vi "utilities_setTimeMode.vi"(8 "error in (no error)":errorcluster, 10 "time column mode (0: Empty)":T1, 11 "data value":T2={"TargetFile"=path "", "StreamMode"=enum."File", "Append?"=FALSE, "ChunkSize"=0, "TimeColumnMode"=enum."Empty", "TimestampFormat"="", "AbsoluteTime?"=FALSE, "FileAttribute "={"Creator"="", "Title"="", "SheetName"=""}, "Column"=[], "FileRef"=refnum, "MemoryRef"=[], "RecordInfo"=[], " ChannelPreviousInfo"=[], "ChannelFirstRecord"=[], "PredefinedFormattedValueLength"=20, "DiskTemplate"={"XMLRef"=[refnum, refnum, refnum, refnum, refnum, refnum], "ZipPath"=path "", "MetaFile"={"Ref"=refnum, "NextRow"=0, "NextPosition"=0, "Block"=[]}, "TempFolder"=path ""}}) -> (0 "error out":errorcluster, 3 "data value out":T2={"TargetFile"=path "", "StreamMode"=enum."File", "Append?"=FALSE, "ChunkSize"=0, "TimeColumnMode"=enum."Empty", "TimestampFormat"="", "AbsoluteTime?"=FALSE, "FileAttribute "={"Creator"="", "Title"="", "SheetName"=""}, "Column"=[], "FileRef"=refnum, "MemoryRef"=[], "RecordInfo"=[], " ChannelPreviousInfo"=[], "ChannelFirstRecord"=[], "PredefinedFormattedValueLength"=20, "DiskTemplate"={"XMLRef"=[refnum, refnum, refnum, refnum, refnum, refnum], "ZipPath"=path "", "MetaFile"={"Ref"=refnum, "NextRow"=0, "NextPosition"=0, "Block"=[]}, "TempFolder"=path ""}})   [LabVIEW 2020, in "NI_ExcelFile.lvlib"]
uses:
  <vilib>/express/express shared/NI_ExcelFile/NI_ExcelFile.lvlib
  <vilib>/express/express shared/NI_ExcelFile/Ctrls/MainData.ctl
  <vilib>/express/express shared/NI_ExcelFile/Ctrls/StreamMode.ctl
  <vilib>/express/express shared/NI_ExcelFile/Ctrls/TimeColumnMode.ctl
  <vilib>/express/express shared/NI_ExcelFile/Ctrls/FileAttribute.ctl
  <vilib>/express/express shared/NI_ExcelFile/Ctrls/Columns.ctl
  <vilib>/express/express shared/NI_ExcelFile/Ctrls/ColumnInfo.ctl
  <vilib>/express/express shared/NI_ExcelFile/Ctrls/DataType.ctl
  <vilib>/express/express shared/NI_ExcelFile/Ctrls/wd_recordInfo.ctl
  <vilib>/express/express shared/NI_ExcelFile/Ctrls/disk_TemplateFile.ctl
  <vilib>/express/express shared/NI_ExcelFile/Ctrls/meta_file.ctl
  <vilib>/express/express shared/NI_ExcelFile/Ctrls/meta_Block.ctl
  <vilib>/express/express shared/NI_ExcelFile/Ctrls/meta_BlockType.ctl
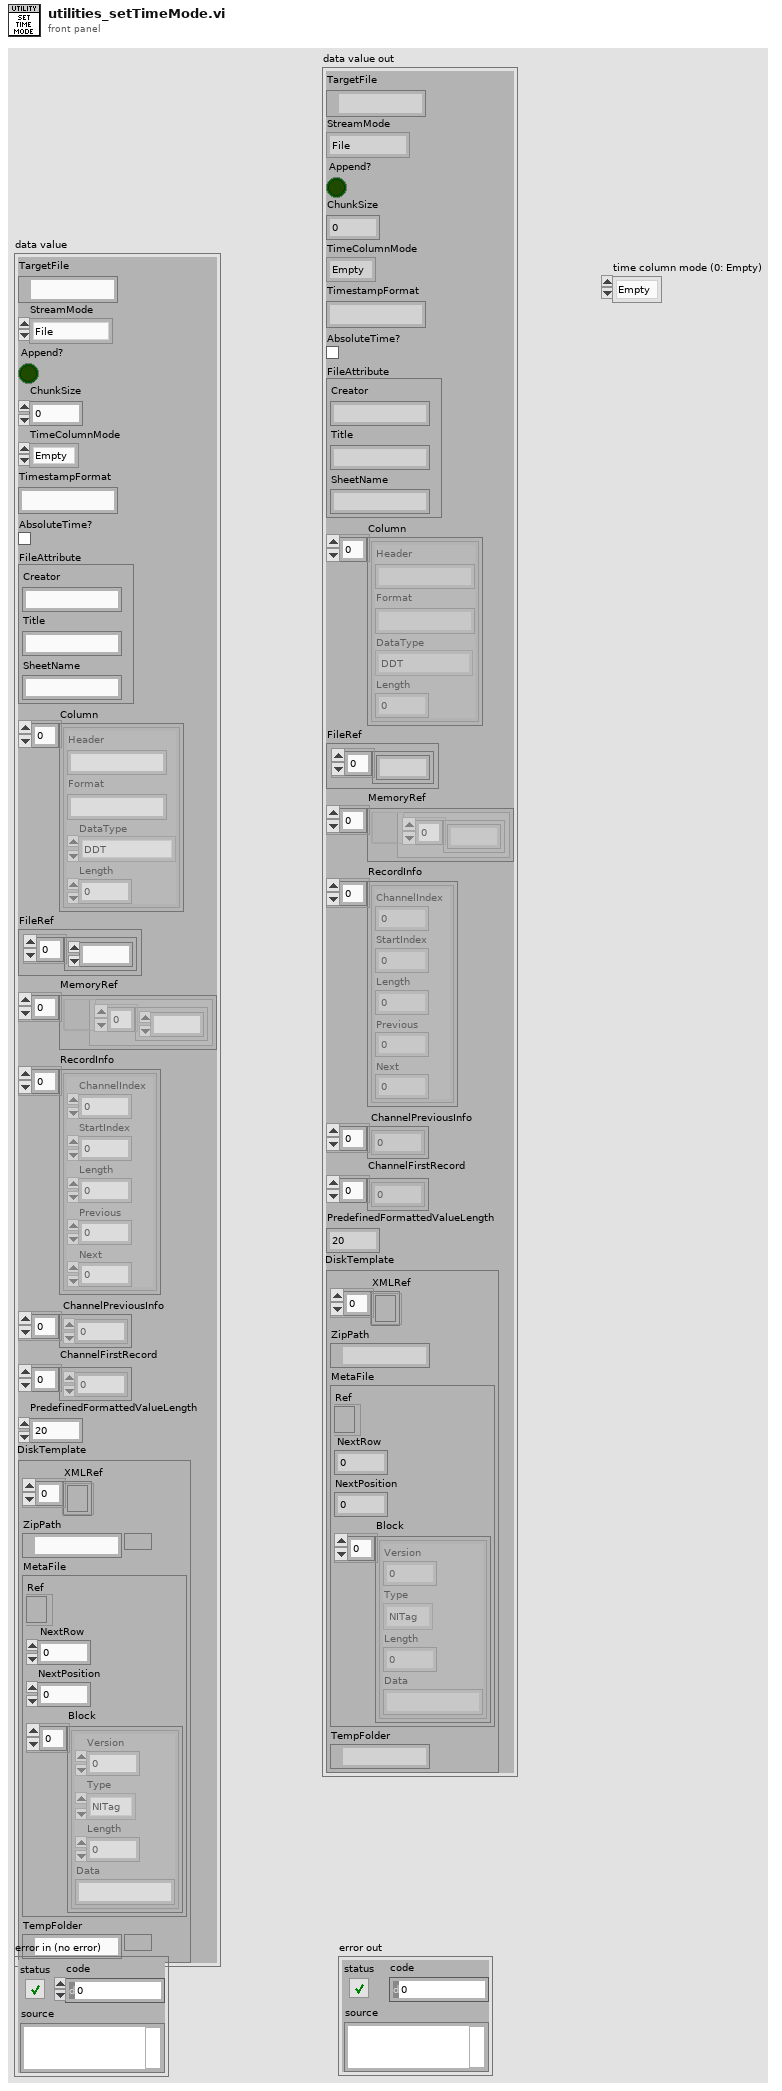
[diagram p1: front panel]
types:
  T1 = typedef "NI_ExcelFile.lvlib/TimeColumnMode.ctl" = enum16{"Empty", "OnePerCh", "One"}
  T2 = typedef "NI_ExcelFile.lvlib/MainData.ctl" = cluster{"TargetFile":path, "StreamMode":T3, "Append?":bool, "ChunkSize":u64, "TimeColumnMode":T1, "TimestampFormat":string, "AbsoluteTime?":bool, "FileAttribute ":T4, "Column":T5, "FileRef":refnum<k1>, "MemoryRef":refnum<data-value>[], "RecordInfo":T8[], " ChannelPreviousInfo":u32[], "ChannelFirstRecord":u32[], "PredefinedFormattedValueLength":i64, "DiskTemplate":T9}
  T3 = typedef "NI_ExcelFile.lvlib/StreamMode.ctl" = enum16{"File", "Memory"}
  T4 = typedef "NI_ExcelFile.lvlib/FileAttribute.ctl" = cluster{"Creator":string, "Title":string, "SheetName":string}
  T5 = typedef "NI_ExcelFile.lvlib/Columns.ctl" = T6[]
  T6 = typedef "NI_ExcelFile.lvlib/ColumnInfo.ctl" = cluster{"Header":string, "Format":string, "DataType":T7, "Length":u64}
  T7 = typedef "NI_ExcelFile.lvlib/DataType.ctl" = enum16{"DDT", "WFM", "Array of STR", "Array of DBL", "Array of I8", "Array of I16", "Array of I32", "Array of I64", "Array of SGL", "Array of U8", "Array of U16", "Array of U32", "Array of U64", "Array of Time"}
  T8 = typedef "NI_ExcelFile.lvlib/wd_recordInfo.ctl" = cluster{"ChannelIndex":u32, "StartIndex":u64, "Length":u64, "Previous":i32, "Next":i32}
  T9 = typedef "NI_ExcelFile.lvlib/disk_TemplateFile.ctl" = cluster{"XMLRef":refnum<file>[], "ZipPath":path, "MetaFile":T10, "TempFolder":path}
  T10 = typedef "NI_ExcelFile.lvlib/meta_file.ctl" = cluster{"Ref":refnum<file>, "NextRow":i32, "NextPosition":i64, "Block":T11[]}
  T11 = typedef "NI_ExcelFile.lvlib/meta_Block.ctl" = cluster{"Version":u16, "Type":T12, "Length":i32, "Data":string}
  T12 = typedef "NI_ExcelFile.lvlib/meta_BlockType.ctl" = enum16{"NITag", "File", "Column"}
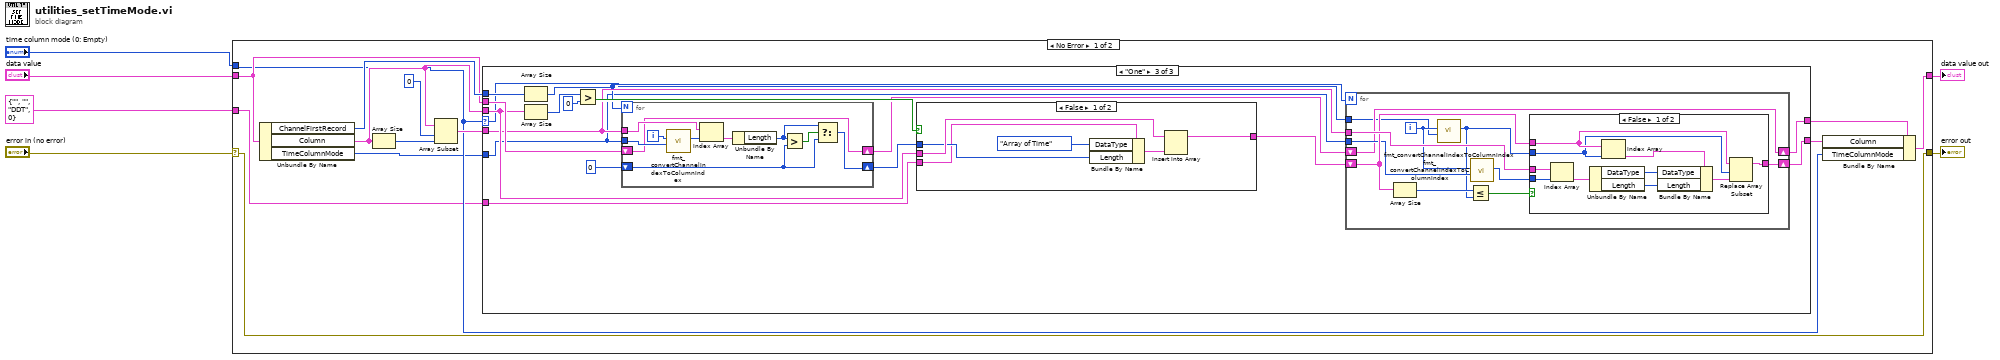
[diagram p0: block diagram]
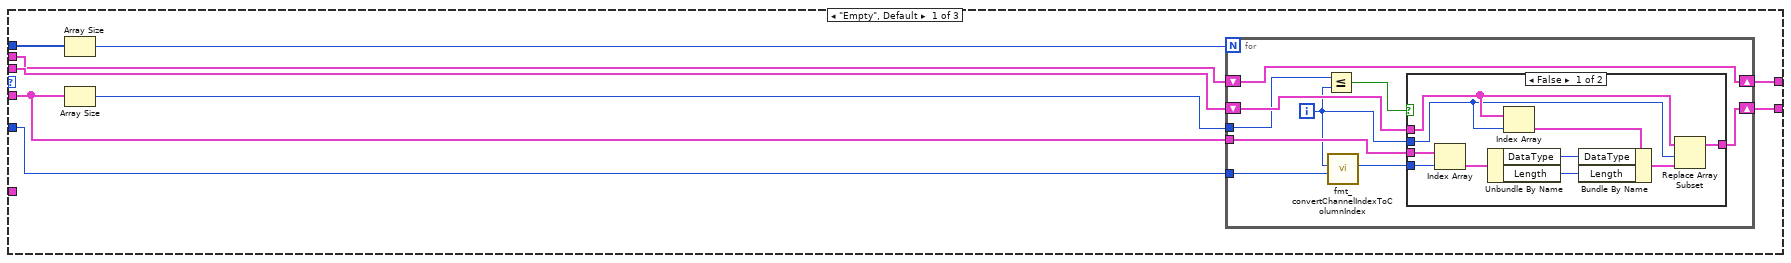
[diagram p2: hidden frame]
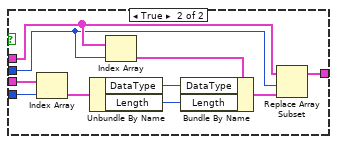
[diagram p3: hidden frame]
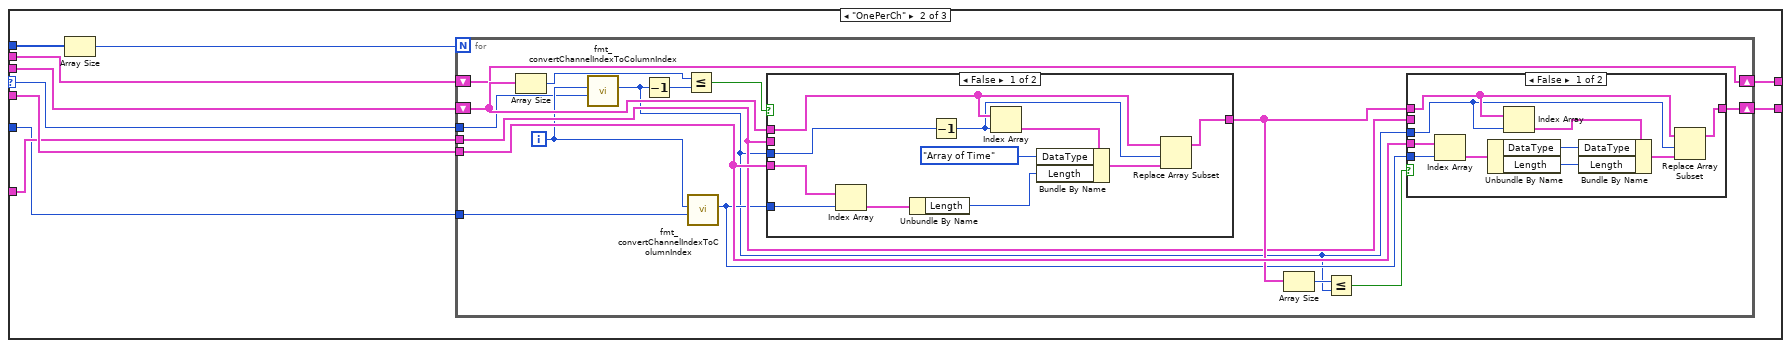
[diagram p4: hidden frame]
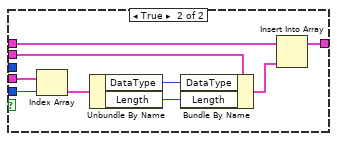
[diagram p5: hidden frame]
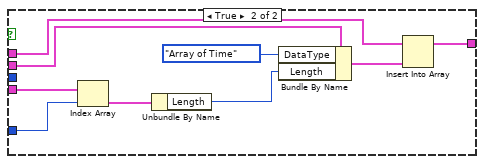
[diagram p6: hidden frame]
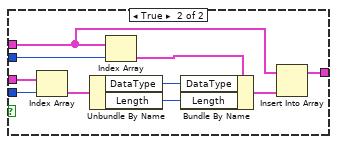
[diagram p7: hidden frame]
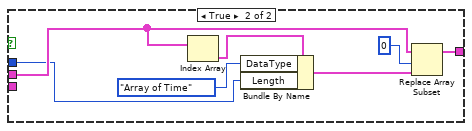
[diagram p8: hidden frame]
diagram:
  n1 = case shown="No Error" "error in (no error)" {
    selector: "error in (no error)" -> [w13 w194]
    tunnel: [w10 w195] -> w4
    tunnel: "data value" -> [w18 w195]
    tunnel: [w13 w194] -> w3
    tunnel: "time column mode (0: Empty)" -> [w9 _]
    tunnel: T6 {"Header"="", "Format"="", "DataType"=enum."DDT", "Length"=0} ("element") -> [w8 _]
    frame No Error {
      n2 = Unbundle By Name(w18) -> ("ChannelFirstRecord"=w19:u32[], "Column"=w16:T5, "TimeColumnMode"=w7:T1)
      n3 = Array Size(array=w16) -> (size(s)=w17:i32)
      n4 = Array Subset(array=w16, index=0, length=w17) -> (w14:T5)
      n5 = case shown="\"One\"" w9 {
        selector: w9 -> [_ w58 w123]
        tunnel: w16 -> [w28 w63 w134]
        tunnel: w19 -> [w23 w67 w130]
        tunnel: w18 -> [w27 w65 w138]
        tunnel: w14 -> [w26 w64 w131]
        tunnel: [w22 w62 w127] -> w12
        tunnel: [w21 w61 w126] -> w11
        tunnel: w8 -> [_ w60 w125]
        tunnel: w7 -> [w20 w59 w124]
        frame "Empty", Default {
          n6 = Array Size(array=w23) -> (size(s)=w24:i32)
          n7 = Array Size(array=w26) -> (size(s)=w25:i32)
          n8 = for {
            N: w24 -> [_]
            tunnel: w26 -> [w35]
            shift-right: [w29] -> w22
            shift-left: w27 -> [w29]
            shift-right: [w34] -> w21
            shift-left: w28 -> [w36]
            tunnel: w25 -> [w33]
            tunnel: w20 -> [w31]
            i -> [w32]
            n9 = Less Or Equal?(x=w33, y=w32) -> (x <= y?=w37:bool)
            n10 = call <vilib>:"fmt_convertChannelIndexToColumnIndex.vi"("TimeColumnMode"=w31, "channel index"=w32) -> ("data column index"=w30:i32)  [unwired: 8 in, 1 out]
            n11 = case shown="False" w37 {
              tunnel: w36 -> [w44 w57]
              tunnel: w32 -> [w43 w54]
              tunnel: w35 -> [w41 w53]
              tunnel: w30 -> [w42 w51]
              tunnel: [w38 w50] -> w34
              frame False {
                n12 = Index Array(array=w41, index=w42) -> (element=w45:T6)
                n13 = Unbundle By Name(w45) -> ("DataType"=w40:T7, "Length"=w39:u64)
                n14 = Index Array(array=w44, index=w43) -> (element=w47:T6)
                n15 = Bundle By Name(cluster=w47, "DataType"=w40, "Length"=w39) -> (w46:T6)
                n16 = Replace Array Subset(array=w44, new element=w46, index=w43) -> (w38:T5)
              }
              frame True {
                n17 = Index Array(array=w53, index=w51) -> (element=w52:T6)
                n18 = Unbundle By Name(w52) -> ("DataType"=w49:T7, "Length"=w48:u64)
                n19 = Index Array(array=w57, index=w54) -> (element=w56:T6)
                n20 = Bundle By Name(cluster=w56, "DataType"=w49, "Length"=w48) -> (w55:T6)
                n21 = Replace Array Subset(array=w57, new element=w55, index=w54) -> (w50:T5)
              }
            }
          }
        }
        frame "OnePerCh" {
          n22 = Array Size(array=w67) -> (size(s)=w66:i32)
          n23 = for {
            N: w66 -> [_]
            tunnel: w64 -> [w80]
            shift-right: [w71] -> w62
            shift-left: w65 -> [w71]
            shift-right: [w76] -> w61
            shift-left: w63 -> [w81]
            tunnel: w59 -> [w73]
            tunnel: w60 -> [w74]
            tunnel: w58 -> [w69]
            i -> [w70]
            n24 = Array Size(array=w81) -> (size(s)=w82:i32)
            n25 = call <vilib>:"fmt_convertChannelIndexToColumnIndex.vi"("TimeColumnMode"=w69, "channel index"=w70) -> ("data column index"=w68:i32)  [unwired: 8 in, 1 out]
            n26 = Decrement(x=w68) -> (x-1=w75:i32)
            n27 = Less Or Equal?(x=w82, y=w75) -> (x <= y?=w83:bool)
            n28 = call <vilib>:"fmt_convertChannelIndexToColumnIndex.vi"("TimeColumnMode"=w73, "channel index"=w70) -> ("data column index"=w72:i32)  [unwired: 8 in, 1 out]
            n29 = case shown="False" w83 {
              tunnel: w81 -> [w110 w122]
              tunnel: w68 -> [w104 _]
              tunnel: w80 -> [w108 w121]
              tunnel: w72 -> [w109 w119]
              tunnel: [w106 w118] -> w79
              tunnel: w74 -> [_ w114]
              frame False {
                n30 = Index Array(array=w108, index=w109) -> (element=w111:T6)
                n31 = Unbundle By Name(w111) -> ("Length"=w107:u64)
                n32 = Decrement(x=w104) -> (x-1=w103:i32)
                n33 = Index Array(array=w110, index=w103) -> (element=w113:T6)
                n34 = Bundle By Name(cluster=w113, "DataType"=DataType."Array of Time" ("Column DataType"), "Length"=w107) -> (w112:T6)
                n35 = Replace Array Subset(array=w110, new element=w112, index=w103) -> (w106:T5)
              }
              frame True {
                n36 = Index Array(array=w121, index=w119) -> (element=w120:T6)
                n37 = Unbundle By Name(w120) -> ("Length"=w117:u64)
                n38 = Bundle By Name(cluster=w114, "DataType"=DataType."Array of Time" ("Column DataType"), "Length"=w117) -> (w115:T6)
                n39 = Insert Into Array(array=w122, new element=w115) -> (w118:T5)  [unwired: 1 in]
              }
            }
            n40 = Array Size(array=w79) -> (size(s)=w78:i32)
            n41 = Less Or Equal?(x=w78, y=w68) -> (x <= y?=w77:bool)
            n42 = case shown="False" w77 {
              tunnel: w79 -> [w90 w102]
              tunnel: w80 -> [w89 w101]
              tunnel: [w87 w99] -> w76
              tunnel: w68 -> [w84 _]
              tunnel: w72 -> [w86 w95]
              tunnel: w74 -> [_ w94]
              frame False {
                n43 = Index Array(array=w89, index=w86) -> (element=w91:T6)
                n44 = Unbundle By Name(w91) -> ("DataType"=w85:T7, "Length"=w88:u64)
                n45 = Index Array(array=w90, index=w84) -> (element=w93:T6)
                n46 = Bundle By Name(cluster=w93, "DataType"=w85, "Length"=w88) -> (w92:T6)
                n47 = Replace Array Subset(array=w90, new element=w92, index=w84) -> (w87:T5)
              }
              frame True {
                n48 = Index Array(array=w101, index=w95) -> (element=w100:T6)
                n49 = Unbundle By Name(w100) -> ("DataType"=w96:T7, "Length"=w98:u64)
                n50 = Bundle By Name(cluster=w94, "DataType"=w96, "Length"=w98) -> (w97:T6)
                n51 = Insert Into Array(array=w102, new element=w97) -> (w99:T5)  [unwired: 1 in]
              }
            }
          }
        }
        frame "One" {
          n52 = Array Size(array=w130) -> (size(s)=w129:i32)
          n53 = Array Size(array=w134) -> (size(s)=w137:i32)
          n54 = Greater?(x=w137, y=0) -> (0:w135:bool)
          n55 = for {
            N: w129 -> [_]
            shift-right: [w188] -> w133
            shift-left: 0 -> [w189]
            shift-right: [w184] -> w128
            shift-left: w138 -> [w184]
            tunnel: w131 -> [w193]
            tunnel: w124 -> [w186]
            i -> [w187]
            n56 = call <vilib>:"fmt_convertChannelIndexToColumnIndex.vi"("TimeColumnMode"=w186, "channel index"=w187) -> ("data column index"=w185:i32)  [unwired: 8 in, 1 out]
            n57 = Index Array(array=w193, index=w185) -> (element=w192:T6)
            n58 = Unbundle By Name(w192) -> ("Length"=w190:u64)
            n59 = Greater?(x=w190, y=w189) -> (0:w191:bool)
            n60 = Select(t=w190, s=w191, f=w189) -> (s? t:f=w188:u64)
          }
          n61 = case shown="False" w135 {
            tunnel: w134 -> [w174 w182]
            tunnel: w133 -> [w172 w179]
            tunnel: [w173 w177] -> w132
            tunnel: w125 -> [w171 _]
            frame False {
              n62 = Bundle By Name(cluster=w171, "DataType"=DataType."Array of Time" ("Column DataType"), "Length"=w172) -> (w175:T6)
              n63 = Insert Into Array(array=w174, new element=w175) -> (w173:T5)  [unwired: 1 in]
            }
            frame True {
              n64 = Index Array(array=w182) -> (element=w181:T6)  [unwired: 1 in]
              n65 = Bundle By Name(cluster=w181, "DataType"=DataType."Array of Time" ("Column DataType"), "Length"=w179) -> (w178:T6)
              n66 = Replace Array Subset(array=w182, new element=w178, index=0) -> (w177:T5)
            }
          }
          n67 = for {
            N: w129 -> [_]
            tunnel: w131 -> [w149]
            shift-right: [w143] -> w127
            shift-left: w128 -> [w143]
            shift-right: [w148] -> w126
            shift-left: w132 -> [w147]
            tunnel: w124 -> [w145]
            tunnel: w123 -> [w141]
            i -> [w142]
            n68 = Array Size(array=w147) -> (size(s)=w146:i32)
            n69 = call <vilib>:"fmt_convertChannelIndexToColumnIndex.vi"("TimeColumnMode"=w141, "channel index"=w142) -> ("data column index"=w140:i32)  [unwired: 8 in, 1 out]
            n70 = Less Or Equal?(x=w146, y=w140) -> (x <= y?=w150:bool)
            n71 = call <vilib>:"fmt_convertChannelIndexToColumnIndex.vi"("TimeColumnMode"=w145, "channel index"=w142) -> ("data column index"=w144:i32)  [unwired: 8 in, 1 out]
            n72 = case shown="False" w150 {
              tunnel: w147 -> [w157 w170]
              tunnel: w140 -> [w156 w167]
              tunnel: w149 -> [w154 w166]
              tunnel: w144 -> [w155 w164]
              tunnel: [w151 w163] -> w148
              frame False {
                n73 = Index Array(array=w154, index=w155) -> (element=w158:T6)
                n74 = Unbundle By Name(w158) -> ("DataType"=w153:T7, "Length"=w152:u64)
                n75 = Index Array(array=w157, index=w156) -> (element=w160:T6)
                n76 = Bundle By Name(cluster=w160, "DataType"=w153, "Length"=w152) -> (w159:T6)
                n77 = Replace Array Subset(array=w157, new element=w159, index=w156) -> (w151:T5)
              }
              frame True {
                n78 = Index Array(array=w166, index=w164) -> (element=w165:T6)
                n79 = Unbundle By Name(w165) -> ("DataType"=w162:T7, "Length"=w161:u64)
                n80 = Index Array(array=w170, index=w167) -> (element=w169:T6)
                n81 = Bundle By Name(cluster=w169, "DataType"=w162, "Length"=w161) -> (w168:T6)
                n82 = Insert Into Array(array=w170, new element=w168) -> (w163:T5)  [unwired: 1 in]
              }
            }
          }
        }
      }
      n83 = Bundle By Name(cluster=w12, "Column"=w11, "TimeColumnMode"=w9) -> (w10:T2)
    }
    frame Error {
    }
  }
  "data value out" <- w4
  "error out" <- w3
